vi "TSCAN_SetSignalValue.vi"(6 "簇":T1, 8 "SigValue":dbl, 9 "Signal":string, 10 "Message":string, 11 "路径输入":path) -> (2 "CANObJ":T1, 3 "路径输出":path)   [LabVIEW 2019]
panel:
  out "tsdb_get_signal_value_can":i32
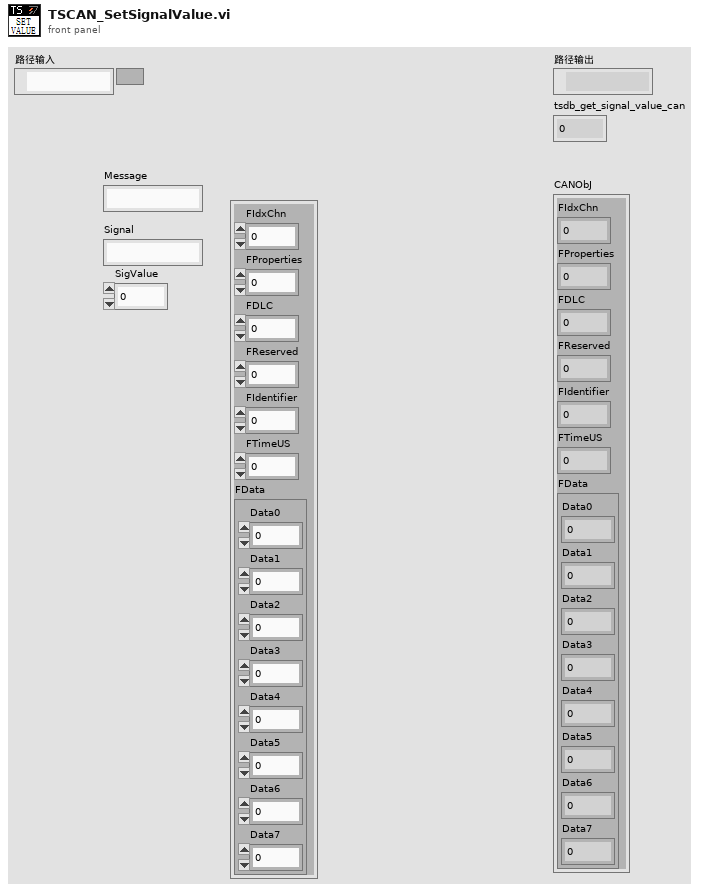
[diagram p1: front panel]
types:
  T1 = cluster{"FIdxChn":u8, "FProperties":u8, "FDLC":u8, "FReserved":u8, "FIdentifier":i32, "FTimeUS":u64, "FData":cluster{"Data0":u8, "Data1":u8, "Data2":u8, "Data3":u8, "Data4":u8, "Data5":u8, "Data6":u8, "Data7":u8}}
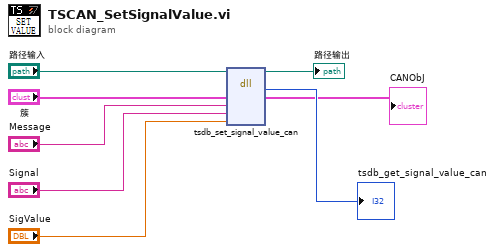
[diagram p0: block diagram]
diagram:
  n1 = dll-call lib="PTH27abs EDemo同星\nTSCAN_V1.0ConfigTSMaster.dll" fn="tsdb_set_signal_value_can"(path in="路径输入", "CANObJ"="簇", "Message"="Message", "Signal"="Signal", "SigValue"="SigValue") -> (path out=→"路径输出":path, "tsdb_get_signal_value_can"=→"tsdb_get_signal_value_can":i32, "CANObJ"=→"CANObJ":T1)  [unwired: 5 in, 1 out]
